vi "Main.vi"() -> ()   [LabVIEW 2017]
doc: "Use this template to build a simple state machine design pattern. Each state executes code and determines which state to transition to."
uses:
  controls/State.ctl
  controls/Data.ctl
  SubPannel/FGV_SubPannel/Func_Subpannel.ctl
  UIchange/GuideTree/FGV_GuideTree.ctl
panel:
  in  "Exit":bool
  out "Msg":string
  in  "Tree":string(tree)
  # "These controls have associated \"Value Changed\" events configured in the Event Structure on the diagram.\n\nReplace them (and reconfigure the Event Structure) with the controls you need for your application."
  # "This template is for the Simple State Machine design pattern.\n\nSee the block diagram for more information on how to use this template."
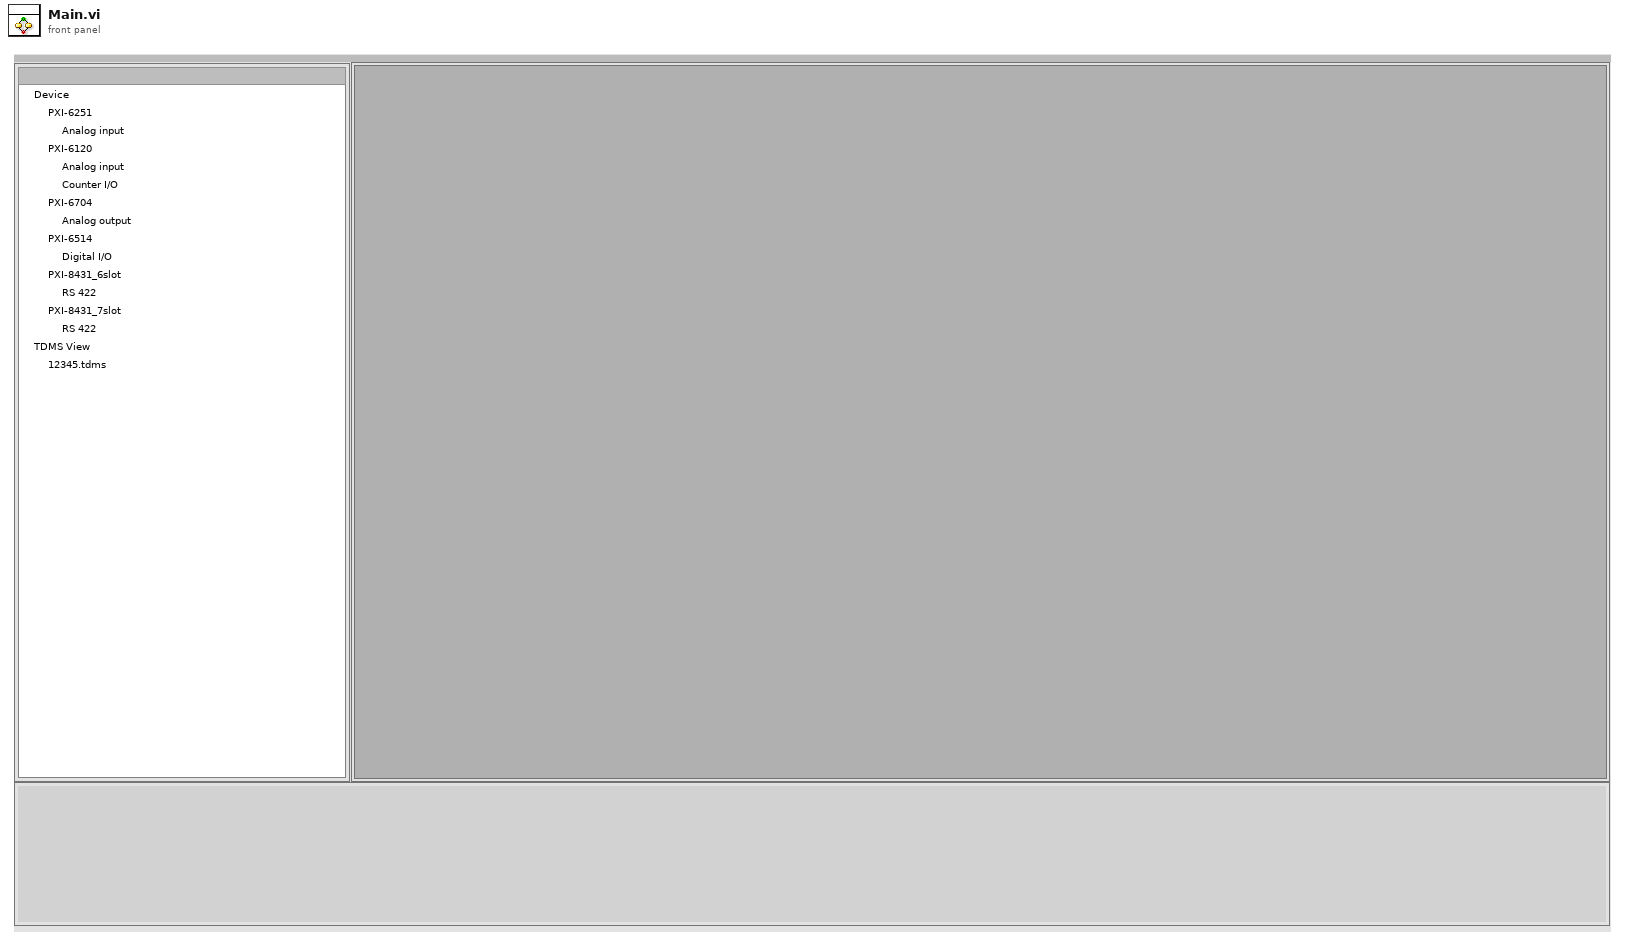
[diagram p1: front panel]
types:
  T1 = typedef "Data.ctl" = cluster{"Boolean <Replace Me>":bool, "String <Replace Me>":string, "Numeric <Replace Me>":dbl, "Main SubPnl":refnum<vi>, "insert VI":refnum<vi>}
  T2 = typedef "State.ctl" = enum16{"Initialize", "Initialize_tree", "Initialize_subpannel", "Wait for Event", "Update SubPannel", "Update State String", "Exit"}
  T3 = typedef "Func_Subpannel.ctl" = enum16{"Initialize", "Get all Opend VIs", "Update Insert VI", "Close all VIs"}
  T4 = typedef "FGV_GuideTree.ctl" = enum16{"SetTree*", "GetTree*", "InitlizeTree", "Get Item infor"}
  T5 = cluster{"Image":path, "Modules":path, "System.ini":path}
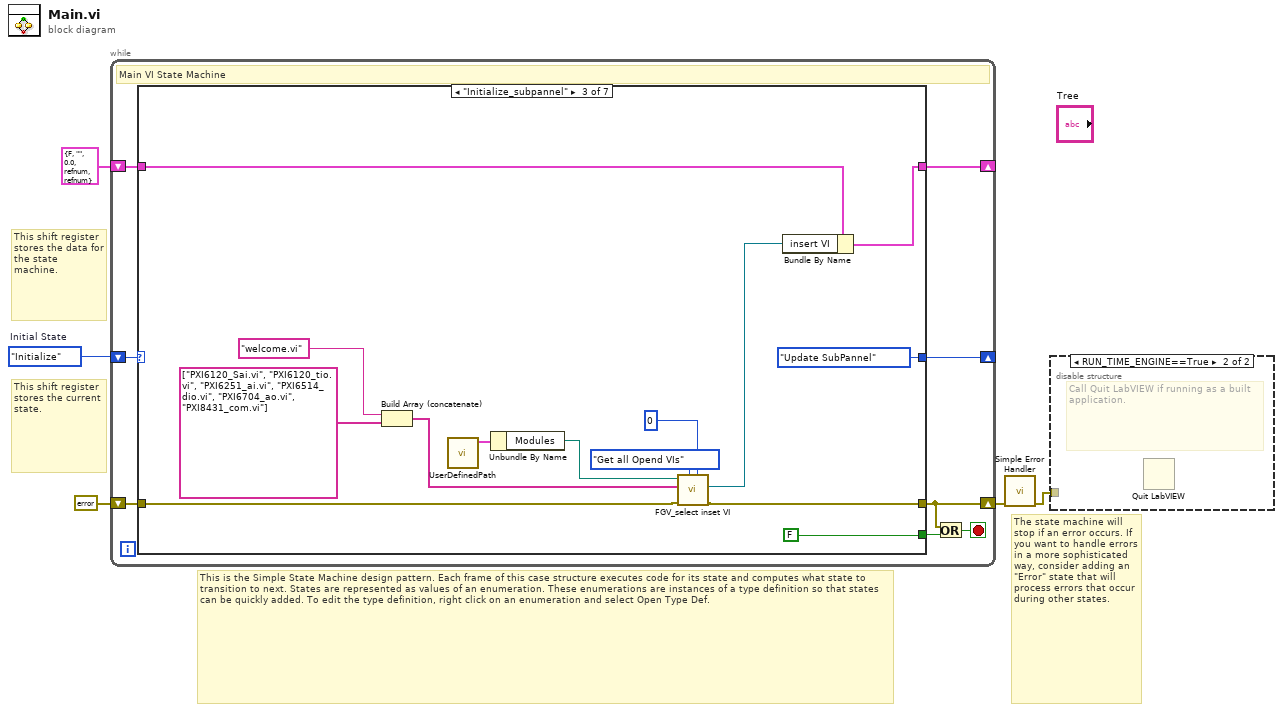
[diagram p0: block diagram]
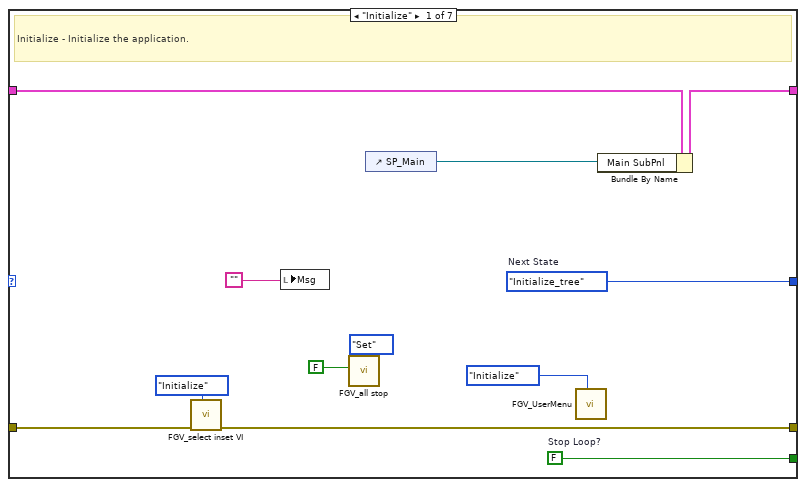
[diagram p3: hidden frame]
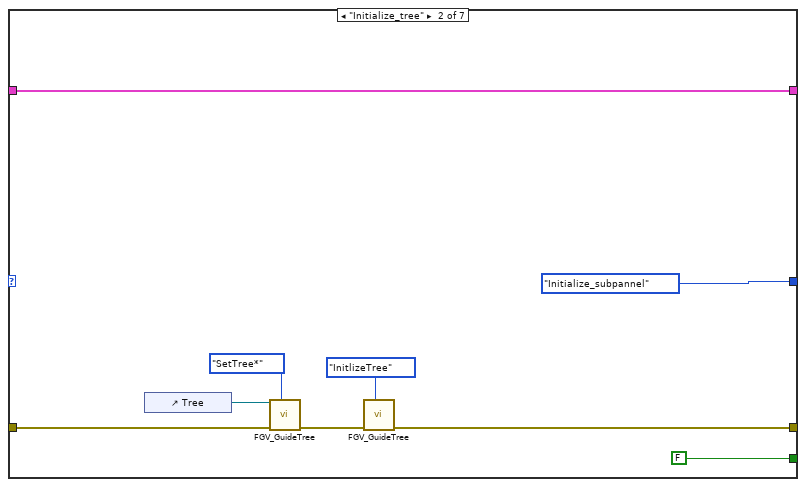
[diagram p4: hidden frame]
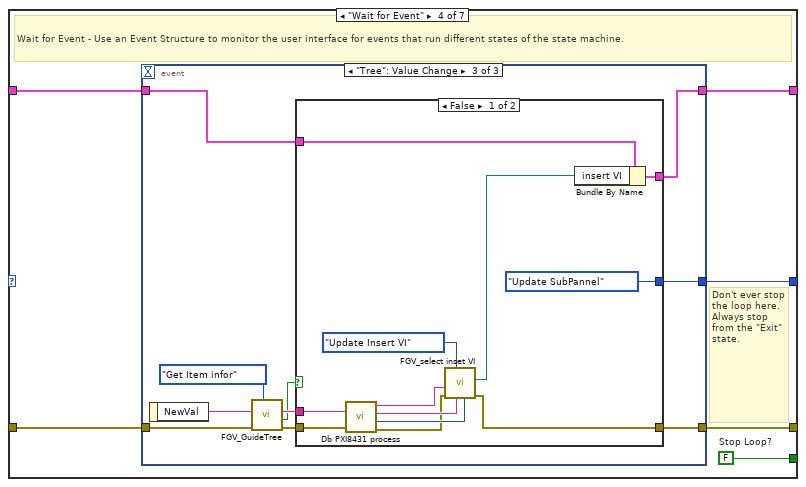
[diagram p5: hidden frame]
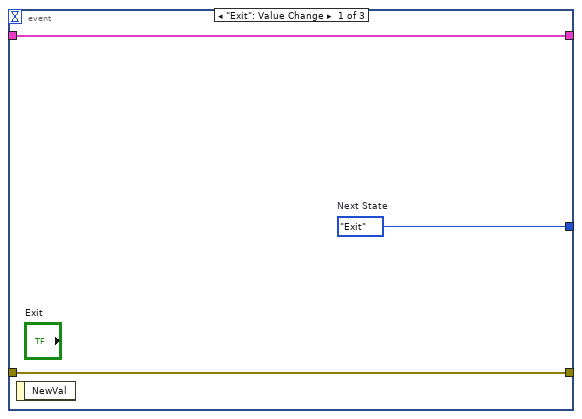
[diagram p6: hidden frame]
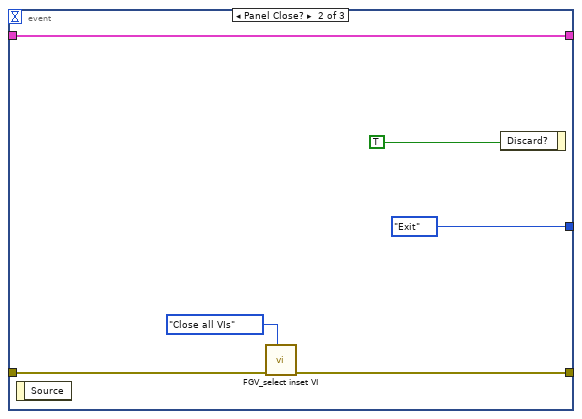
[diagram p7: hidden frame]
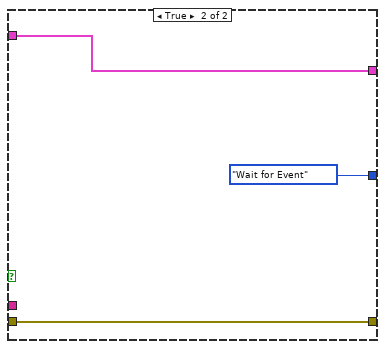
[diagram p8: hidden frame]
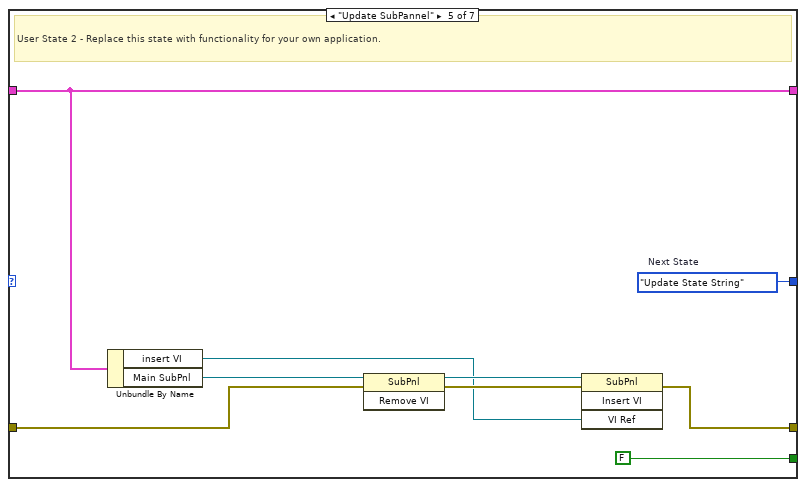
[diagram p9: hidden frame]
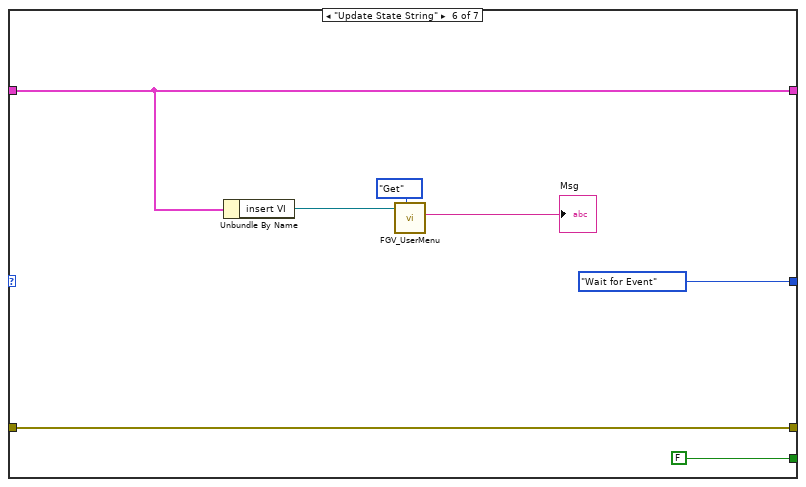
[diagram p10: hidden frame]
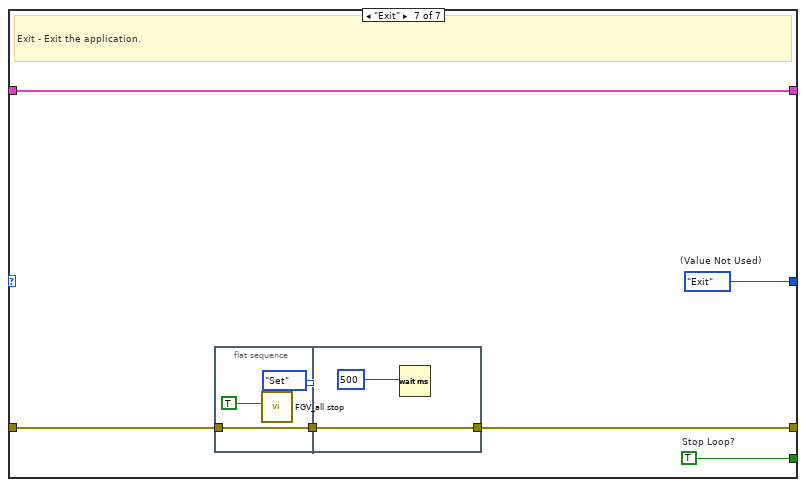
[diagram p11: hidden frame]
diagram:
  w5 = State."Initialize"  # Initial State
  # "The state machine will stop if an error occurs. If you want to handle errors in a more sophisticated way, consider adding an \"Error\" state that will process errors that occur during other states."
  # "This shift register stores the data for the state machine."
  # "This is the Simple State Machine design pattern. Each frame of this case structure executes code for its state and computes what state to transition to next. States are represented as values of an enumeration. These enumerations are instances of a type definition so that states can be quickly added. To edit the type definition, right click on an enumeration and select Open Type Def."
  # "This shift register stores the current state."
  n1 = while {
    shift-right: [w6] -> _
    shift-left: w5 -> [w7]
    shift-right: [w12] -> _
    shift-left: T1 {"Boolean <Replace Me>"=FALSE, "String <Replace Me>"="", "Numeric <Replace Me>"=0.0, "Main SubPnl"=refnum, "insert VI"=refnum} ("Data") -> [w13]
    shift-right: [w8] -> w2
    shift-left: errorcluster {"status"=FALSE, "code"=0, "source"=""} ("error constant") -> [w11]
    stop <- w9 stop-if-true
    # "Main VI State Machine"
    n2 = case shown="\"Initialize_subpannel\"" w7 {
      tunnel: [w25 State."Initialize_subpannel" ("(Value Not Used)") State."Update SubPannel" ("(Value Not Used)") w49 w97 State."Wait for Event" ("(Value Not Used)") w110] -> w6
      tunnel: [w24 FALSE ("Stop Loop?") FALSE w54 FALSE ("Stop Loop?") FALSE ("Stop Loop?") w108] -> w10
      tunnel: w13 -> [w23 w34 w37 w53 w95 w99 w109]
      tunnel: [w22 w34 w36 w52 w95 w99 w109] -> w12
      tunnel: w11 -> [w21 w32 w42 w51 w93 w104 w107]
      tunnel: [w15 w31 w43 w50 w89 w104 w105] -> w8
      frame "Initialize" {
        w24 = FALSE  # Stop Loop?
        w25 = State."Initialize_tree"  # Next State
        # "Initialize - Initialize the application."
        n3 = call "FGV_select inset VI.vi"("Function"=Func_Subpannel."Initialize", "error in (no error)"=w21) -> ("error out"=w15:errorcluster)  [unwired: 8 in, 1 out]
        n4 = local write "Msg"("") -> ()
        n5 = call "FGV_all stop.vi"("Enum"=enum16{"Set", "Get"}."Set", "All Stop"=FALSE) -> ()  [unwired: 9 in, 1 out]
        n6 = control-ref of="SP_Main"() -> (w20:refnum<vi>)
        n7 = call "FGV_UserMenu.vi"("Command"=enum16{"Initialize", "Set", "Get"}."Initialize") -> ()  [unwired: 10 in, 1 out]
        n8 = Bundle By Name(cluster=w23, "Main SubPnl"=w20) -> (w22:T1)
      }
      frame "Initialize_tree" {
        n9 = control-ref of="Tree"() -> (w26:refnum<vi>)
        n10 = call "FGV_GuideTree.vi"("Action"=FGV_GuideTree."SetTree*", "error in"=w32, "Tree*"=w26) -> ("error out"=w28:errorcluster)  [unwired: 5 in, 3 out]
        n11 = call "FGV_GuideTree.vi"("Action"=FGV_GuideTree."InitlizeTree", "error in"=w28) -> ("error out"=w31:errorcluster)  [unwired: 6 in, 3 out]
      }
      frame "Initialize_subpannel" {
        n12 = Build Array (concatenate)("welcome.vi", string[] ["PXI6120_Sai.vi", "PXI6120_tio.vi", "PXI6251_ai.vi", "PXI6514_dio.vi", "PXI6704_ao.vi", "PXI8431_com.vi"]) -> (w39:string[])
        n13 = call "UserDefinedPath.vi"() -> ("ProDefPath"=w46:T5)  [unwired: 11 in]
        n14 = Unbundle By Name(w46) -> ("Modules"=w40:path)
        n15 = call "FGV_select inset VI.vi"("First Run"=0, "Function"=Func_Subpannel."Get all Opend VIs", "error in (no error)"=w42, "VIs Name"=w39, "ModulesPath"=w40) -> ("error out"=w43:errorcluster, "Inset VI"=w35:refnum<vi>)  [unwired: 5 in]
        n16 = Bundle By Name(cluster=w37, "insert VI"=w35) -> (w36:T1)
      }
      frame "Wait for Event" {
        w54 = FALSE  # Stop Loop?
        # "Don't ever stop the loop here. Always stop from the \"Exit\" state."
        # "Wait for Event - Use an Event Structure to monitor the user interface for events that run different states of the state machine."
        n17 = event shown="[2] \"Tree\": Value Change" {
          selector: _ -> [_ _ _]
          dyn-events: _ -> [_ _ _]
          timeout: _ -> [_ _ _]
          tunnel: w53 -> [w57 w63 w68]
          tunnel: [w57 w63 w72] -> w52
          tunnel: w51 -> [w56 w62 w71]
          tunnel: [w56 w59 w64] -> w50
          tunnel: [w55 State."Exit" ("Next State") w73] -> w49
          event "Exit": Value Change {
            w55 = State."Exit"  # Next State
            n18 = event-data() -> ()  [unwired: 1 in, 1 out]
          }
          event Panel Close? {
            n19 = event-data() -> ()  [unwired: 1 in, 1 out]
            n20 = call "FGV_select inset VI.vi"("Function"=Func_Subpannel."Close all VIs", "error in (no error)"=w62) -> ("error out"=w59:errorcluster)  [unwired: 8 in, 1 out]
            n21 = event-data("Discard?"=TRUE) -> ()  [unwired: 1 in, 1 out]
          }
          event "Tree": Value Change {
            n22 = event-data() -> ("NewVal"=w69:string)  [unwired: 1 in]
            n23 = call "FGV_GuideTree.vi"("Action"=FGV_GuideTree."Get Item infor", "error in"=w71, "Tag"=w69) -> ("error out"=w67:errorcluster, "No Subpunnel"=w65:bool, "UIname"=w66:string)  [unwired: 5 in, 1 out]
            n24 = case shown="False" w65 {
              tunnel: [State."Update SubPannel" ("Next State") State."Wait for Event" ("Next State")] -> w73
              tunnel: [w84 w88] -> w72
              tunnel: w68 -> [w83 w88]
              tunnel: w67 -> [w77 w86]
              tunnel: w66 -> [w76 _]
              tunnel: [w75 w86] -> w64
              frame False {
                n25 = call "Db PXI8431 process.vi"("error in (no error)"=w77, "UIname"=w76) -> ("error out"=w74:errorcluster, "Value"=w78:i32, "Parameter"=w79:string, "Insert VI"=w80:string)  [unwired: 6 in]
                n26 = call "FGV_select inset VI.vi"("Value"=w78, "Parameter"=w79, "Function"=Func_Subpannel."Update Insert VI", "error in (no error)"=w74, "Inser VI name"=w80) -> ("error out"=w75:errorcluster, "Inset VI"=w81:refnum<vi>)  [unwired: 5 in]
                n27 = Bundle By Name(cluster=w83, "insert VI"=w81) -> (w84:T1)
              }
              frame True {
              }
            }
          }
        }
      }
      frame "Update SubPannel" {
        w97 = State."Update State String"  # Next State
        # "User State 2 - Replace this state with functionality for your own application."
        n28 = Unbundle By Name(w95) -> ("insert VI"=w90:refnum<vi>, "Main SubPnl"=w94:refnum<vi>)
        n29 = invoke class="SubPnl" method="Remove VI"(reference=w94, error in=w93) -> (reference out=w92:refnum<vi>, error out=w91:errorcluster)  [unwired: 1 in, 1 out]
        n30 = invoke class="SubPnl" method="Insert VI"(reference=w92, error in=w91, "VI Ref"=w90) -> (error out=w89:errorcluster)  [unwired: 1 in, 3 out]
      }
      frame "Update State String" {
        n31 = Unbundle By Name(w99) -> ("insert VI"=w98:refnum<vi>)
        n32 = call "FGV_UserMenu.vi"("Command"=enum16{"Initialize", "Set", "Get"}."Get", "VI Refnum"=w98) -> ("String"=→"Msg":string)  [unwired: 9 in]
      }
      frame "Exit" {
        w108 = TRUE  # Stop Loop?
        w110 = State."Exit"  # (Value Not Used)
        # "Exit - Exit the application."
        n33 = flat-sequence {
          tunnel: w107 -> [w111]
          tunnel: [w111] -> w106
          tunnel: [w114] -> w105
          tunnel: w106 -> [w114]
          frame #0 {
            n34 = call "FGV_all stop.vi"("Enum"=enum16{"Set", "Get"}."Set", "All Stop"=TRUE) -> ()  [unwired: 9 in, 1 out]
          }
          frame #1 {
            n35 = Wait (ms)(milliseconds to wait=500) -> ()  [unwired: 1 out]
          }
        }
      }
    }
    n36 = Or(x=w8, y=w10) -> (x .or. y?=w9:bool)
  }
  n37 = call <vilib>:"Simple Error Handler.vi"("error in (no error)"=w2) -> ("error out"=w1:errorcluster)  [unwired: 4 in, 4 out]
  n38 = disable-structure shown="RUN_TIME_ENGINE==True" {
    disable-tunnel: w1 -> [_ _]
    frame condition #0 (active) {
    }
    frame condition #1 {
      # "Call Quit LabVIEW if running as a built application."
      n39 = Quit LabVIEW() -> ()  [unwired: 1 in]
    }
  }
